vi "Calc Allan variance.vi"(8 "error in":errorcluster, 10 "taus":sgl[](array[numeric]), 11 "CRDS Cell in":refnum<class "CRDS Cell.lvclass">) -> (0 "error out":errorcluster, 3 "CRDS Cell out":refnum<class "CRDS Cell.lvclass">)   [LabVIEW 2014, in "CRDS Lib.lvlib" / "CRDS Cell.lvclass"]
uses:
  CRDS Cell.lvclass
  CRDS Cell.lvclass/CRDS Cell.ctl
  Data/Cell/CRDS Cell Data.lvclass/CRDS Cell Data.ctl
  Data/Cell/Write Allan Variances.vi
  General/Math Utilities.lvlib
  Data/Cell/CRDS Cell Data.lvclass
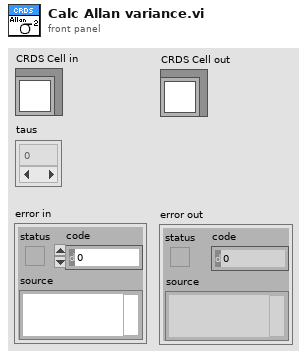
[diagram p1: front panel]
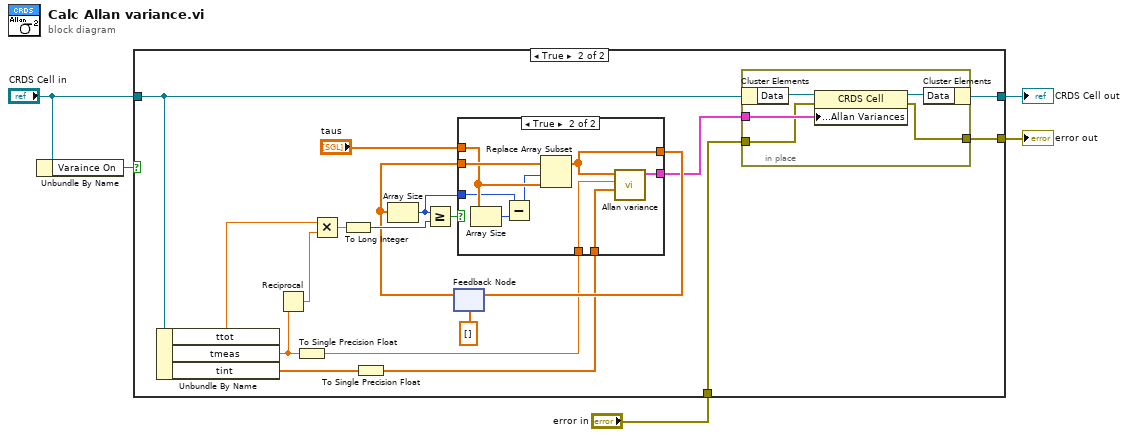
[diagram p0: block diagram]
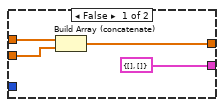
[diagram p3: hidden frame]
diagram:
  n1 = Unbundle By Name("CRDS Cell in") -> ("Varaince On"=w2:bool)
  n2 = case shown="True" w2 {
    tunnel: [w6 w15] -> w5
    tunnel: [w7 w14] -> w4
    tunnel: "CRDS Cell in" -> [w7 w13]
    tunnel: "error in" -> [w6 w12]
    frame False {
    }
    frame True {
      n3 = Unbundle By Name(w13) -> ("ttot"=w25:dbl, "tmeas"=w11:dbl, "tint"=w9:sgl[])
      n4 = Reciprocal(x=w11) -> (1/x=w26:dbl)
      n5 = To Single Precision Float(number=w11) -> (single precision float=w10:sgl)
      n6 = Multiply(x=w25, y=w26) -> (x*y=w23:dbl)
      n7 = To Long Integer(number=w23) -> (32bit integer=w22:i32)
      n8 = To Single Precision Float(number=w9) -> (single precision float=w8:sgl[])
      n9 = feedback #1(sgl[] [] ("taus")) -> (w19:sgl[])
      n10 = Array Size(array=w19) -> (size(s)=w17:i32)
      n11 = Greater Or Equal?(x=w17, y=w22) -> (x >= y?=w21:bool)
      n12 = case shown="True" w21 {
        tunnel: w10 -> [_ w44]
        tunnel: w8 -> [_ w43]
        tunnel: "taus" -> [w35 w41]
        tunnel: w19 -> [w34 w42]
        tunnel: [w33 w37] -> w18
        tunnel: w17 -> [_ w39]
        tunnel: [cluster{"iTime":sgl[], sgl[]} {"iTime"=[], []} ("Allan Variances") w36] -> w16
        frame False {
          n13 = Build Array (concatenate)(w35, w34) -> (w33:sgl[])
        }
        frame True {
          n14 = Array Size(array=w41) -> (size(s)=w40:i32)
          n15 = Subtract(x=w39, y=w40) -> (x-y=w38:i32)
          n16 = Replace Array Subset(array=w42, new element=w41, index=w38) -> (w37:sgl[])
          n17 = call "Allan variance.vi"("iTime"=w43, "mTime"=w44, "Data In"=w37) -> ("Allan Variances"=w36:cluster{"iTime":sgl[], sgl[]})  [unwired: 8 in]
        }
      }
      n18 = feedback-in #1(w18) -> ()
      n19 = in-place {
        in-place-border: w16 -> [w30]
        in-place-border: w12 -> [w29]
        in-place-border: [w28] -> w15
        n20 = in-place-cluster #2(w13) -> ("Data"=w31:refnum<class "CRDS Cell Data.lvclass">)
        n21 = property class="CRDS Cell"(reference=w31, error in=w29, "Data Access:Allan Variances"=w30) -> (reference out=w27:refnum<class "CRDS Cell Data.lvclass">, error out=w28:errorcluster)
        n22 = in-place-cluster #2("Data"=w27) -> (w14:refnum<class "CRDS Cell.lvclass">)
      }
    }
  }
  "error out" <- w5
  "CRDS Cell out" <- w4
